vi "closeMeas.vi"(8 "error in (no error)":errorcluster, 11 "FPGA VI (in) 2":T1) -> ()   [LabVIEW 2021]
uses:
  <vilib>/rvi/interface/nirviCloseFPGA/nirviCloseFPGA.xnode
  acdc-PV-emulators/FPGA Bitfiles/FPGA.ctl
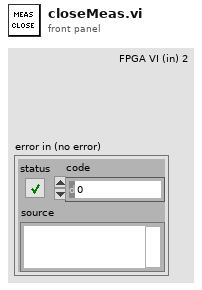
[diagram p1: front panel]
types:
  T1 = typedef "FPGA.ctl" = refnum<k20>
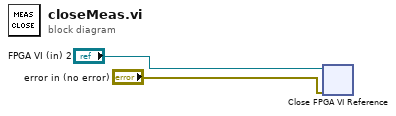
[diagram p0: block diagram]
diagram:
  n1 = xnode "Close FPGA VI Reference"("FPGA VI Reference In"="FPGA VI (in) 2", "error in"="error in (no error)") -> ()  [unwired: 1 out]
